vi "Save into DOM XML.vi"(8 "Error In":errorcluster, 9 "Save UIP List (True)":bool=TRUE, 10 "DOM In":refnum<k20>, 11 "UIM In":refnum<data-value>) -> (0 "Error Out":errorcluster, 2 "DOM Out":refnum<k20>, 3 "UIM Out":refnum<data-value>)   [LabVIEW 2020, in "UIM.lvlib" / "UIM.lvclass"]
doc: "Internal function only."
uses:
  UIM.lvclass
  UIM.lvclass/UIM.ctl
  UIP Interface/UIP Interface.lvclass
  <vilib>/xml/Close Reference(Node).vi
  <vilib>/xml/NI_XML.lvlib
  <resource>/objmgr/DOMUserDefRef.rc
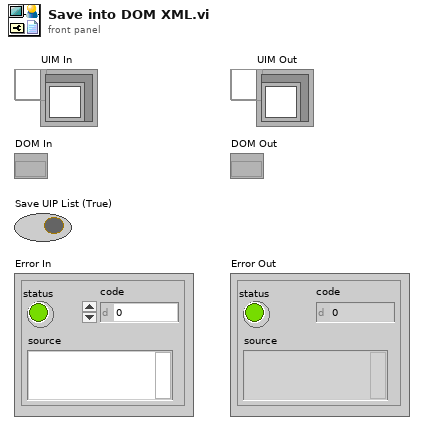
[diagram p1: front panel]
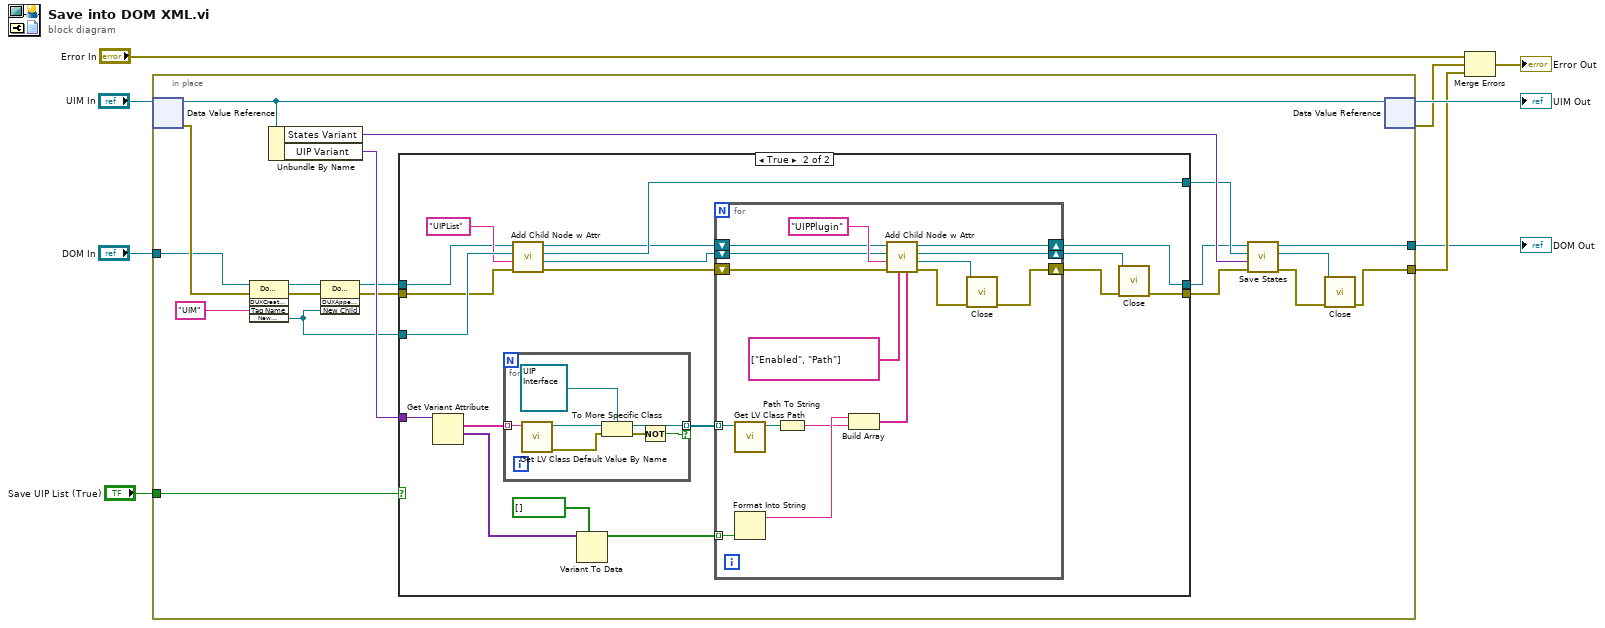
[diagram p0: block diagram]
diagram:
  n1 = in-place {
    in-place-border: [w22] -> w5
    in-place-border: "DOM In" -> [w10]
    in-place-border: [w21] -> w2
    in-place-border: "Save UIP List (True)" -> [w19]
    n2 = in-place-dvr #1("UIM In") -> (w28:refnum<class "UIM.lvclass">, w27:errorcluster)
    n3 = invoke class="Document" method="DUXCreateElement"(reference=w10, error in=w27, "Tag Name"="UIM") -> (reference out=w14:refnum<k20>, error out=w15:errorcluster, "New Element"=w12:refnum<k20>)  [unwired: 2 in, 2 out]
    n4 = Unbundle By Name(w28) -> ("States Variant"=w25:variant, "UIP Variant"=w20:variant)
    n5 = invoke class="Document" method="DUXAppendChild"(reference=w14, error in=w15, "New Child"=w12) -> (reference out=w13:refnum<k20>, error out=w11:errorcluster)  [unwired: 1 in, 2 out]
    n6 = case shown="True" w19 {
      tunnel: w20 -> [_ w46]
      tunnel: w11 -> [w30 w32]
      tunnel: w13 -> [w29 w33]
      tunnel: [w29 w43] -> w16
      tunnel: w12 -> [w31 w42]
      tunnel: [w30 w39] -> w17
      tunnel: [w31 w38] -> w18
      frame False {
      }
      frame True {
        n7 = Get Variant Attribute(Variant=w46) -> (names=w48:string[], values=w47:variant[])  [unwired: 3 in, 2 out]
        n8 = for {
          tunnel: w48 -> [w72] mode=indexing
          tunnel: [w68] -> w45 mode=indexing if=w66
          n9 = call <vilib>:"Get LV Class Default Value By Name.vi"("class name"=w72) -> ("error out"=w69:errorcluster, "object"=w71:refnum<class>)  [unwired: 9 in]
          n10 = To More Specific Class(target class=refnum<class "UIP Interface.lvclass"> refnum ("UIP"), reference=w71, error in=w69) -> (specific class reference=w68:refnum<class "UIP Interface.lvclass">, error out=w67:errorcluster)
          n11 = Not(x=w67) -> (.not. x?=w66:bool)
        }
        n12 = call "Add Child Node w Attr.vi"("Error In"=w32, "Tag Name"="UIPList", "Parent Node"=w42, "DOM In"=w33) -> ("Error Out"=w34:errorcluster, "Child Node"=w37:refnum<k20>, "Parent Node"=w38:refnum<k20>, "DOM Out"=w36:refnum<k20>)  [unwired: 4 in]
        n13 = Variant To Data(type=bool[] [], Variant=w47) -> (data=w44:bool[])  [unwired: 1 in, 1 out]
        n14 = for {
          shift-right: [w62] -> w40
          shift-left: w37 -> [w63]
          shift-right: [w60] -> w43
          shift-left: w36 -> [w61]
          shift-right: [w57] -> w41
          shift-left: w34 -> [w64]
          tunnel: w45 -> [w55] mode=indexing
          tunnel: w44 -> [w54] mode=indexing
          n15 = call <vilib>:"Get LV Class Path.vi"("object"=w55) -> ("class path"=w52:path)  [unwired: 9 in, 1 out]
          n16 = Format Into String(w54) -> (resulting string=w53:string)  [unwired: 3 in, 1 out]
          n17 = Path To String(path=w52) -> (string=w51:string)
          n18 = Build Array(w53, w51) -> (w50:string[])
          n19 = call "Add Child Node w Attr.vi"("Values"=w50, "Names"=string[] ["Enabled", "Path"], "Error In"=w64, "Tag Name"="UIPPlugin", "Parent Node"=w63, "DOM In"=w61) -> ("Error Out"=w58:errorcluster, "Child Node"=w59:refnum<k20>, "Parent Node"=w62:refnum<k20>, "DOM Out"=w60:refnum<k20>)  [unwired: 2 in]
          n20 = call-poly <vilib>:"Close.vi"("error in (no error)"=w58, "node"=w59) -> ("error out"=w57:errorcluster)  [unwired: 7 in]
        }
        n21 = call-poly <vilib>:"Close.vi"("error in (no error)"=w41, "node"=w40) -> ("error out"=w39:errorcluster)  [unwired: 7 in]
      }
    }
    n22 = call "Save States.vi"("Error In"=w17, "States Variant"=w25, "UIM Tag"=w18, "XML Refnum"=w16) -> ("XML Error Out"=w23:errorcluster, "UIM Tag Out"=w24:refnum<k20>, "XML Refnum Out"=w21:refnum<k20>)  [unwired: 5 in]
    n23 = call-poly <vilib>:"Close.vi"("error in (no error)"=w23, "node"=w24) -> ("error out"=w22:errorcluster)  [unwired: 7 in]
    n24 = in-place-dvr #1(w28) -> (→"UIM Out":refnum<data-value>, w4:errorcluster)
  }
  "DOM Out" <- w2
  n25 = Merge Errors("Error In", w4, w5) -> (→"Error Out":errorcluster)
